vi "PathPlanner_Waypoint_AutoCtrlPoints.vi"(4 "NextExists":bool, 6 "PrevExists":bool, 8 "NextAnchor":T2 {"Y" format="%14.3f"; "X" format="%14.3f"}, 9 "PrevAnchor":T2 {"Y" format="%14.3f"; "X" format="%14.3f"}, 10 "Heading":T1={"VALUE"=0.0, "COS"=1.0, "SIN"=0.0} {"SIN" format="%13.4f"; "COS" format="%13.4f"; "VALUE" format="%13.4f"}, 11 "Anchor":T2 {"Y" format="%14.3f"; "X" format="%14.3f"}) -> (3 "Waypoint":T3 {"nextControl"."Y" format="%14.3f"; "nextControl"."X" format="%14.3f"; "anchor"."Y" format="%14.3f"; "anchor"."X" format="%14.3f"; "prevControl"."Y" format="%14.3f"; "prevControl"."X" format="%14.3f"})   [LabVIEW 2019, in "PathPlanner24.lvlib"]
doc: "Convert bezier points to waypoints allowing them to be written to a JSON string.\n\nInputs: \n - Bezier - array of translation2s - List of bezier points\n\nOutputs:\n - waypoints - array of cluster - waypoints compatible with pathplanner path JSON strings."
uses:
  PathPlanner24.lvlib
  TypeDef/PathPlannerWaypoint.ctl
  <vilib>/Rock Robotics/WPI/ThirdParty/JAS_Junk/TrajLib/TypeDef/TRANSLATION2D.ctl
  <vilib>/Rock Robotics/WPI/ThirdParty/JAS_Junk/TrajLib/Trajectory_Library.lvlib
  <vilib>/Rock Robotics/WPI/ThirdParty/JAS_Junk/TrajLib/TypeDef/ROTATION2D.ctl
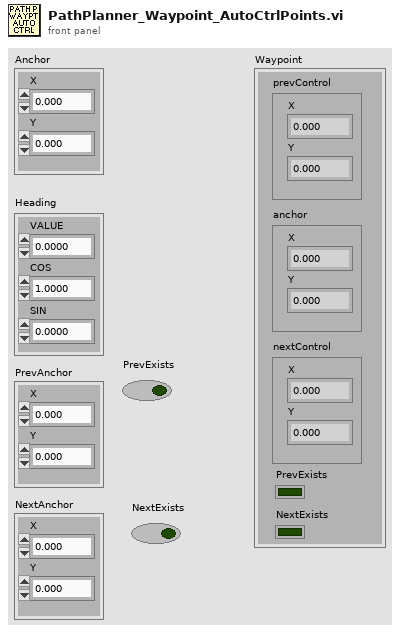
[diagram p1: front panel]
types:
  T1 = typedef "Trajectory_Library.lvlib/ROTATION2D.ctl" = cluster{"VALUE":dbl, "COS":dbl, "SIN":dbl}
  T2 = typedef "Trajectory_Library.lvlib/TRANSLATION2D.ctl" = cluster{"X":dbl, "Y":dbl}
  T3 = typedef "PathPlanner24.lvlib/PathPlannerWaypoint.ctl" = cluster{"prevControl":T2, "anchor":T2, "nextControl":T2, "PrevExists":bool, "NextExists":bool}
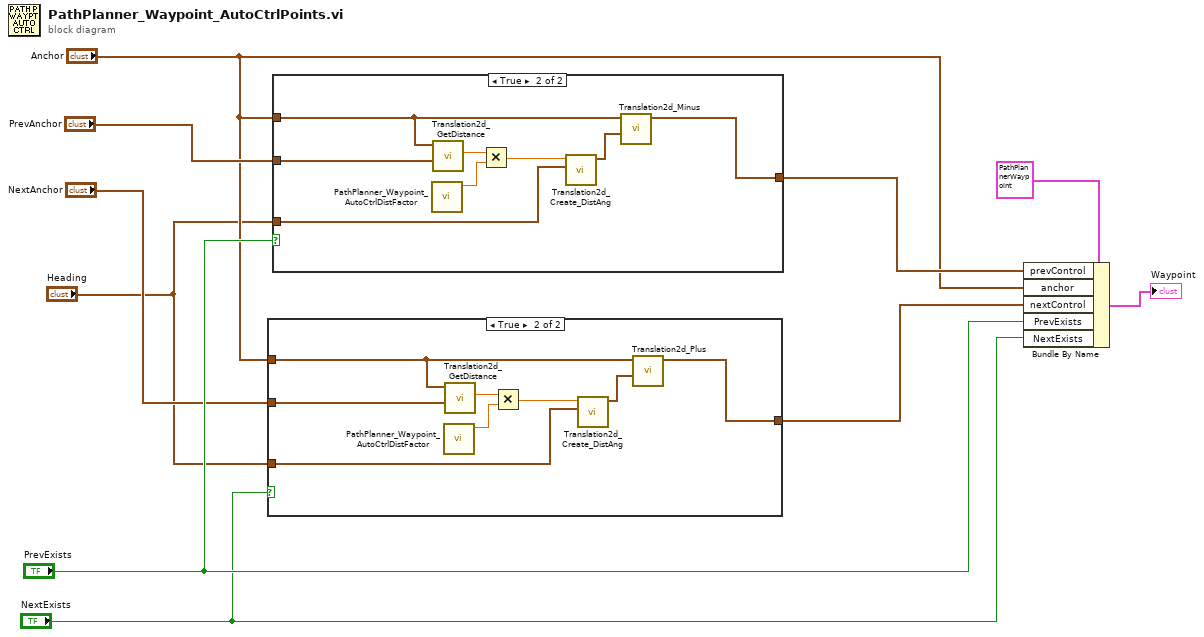
[diagram p0: block diagram]
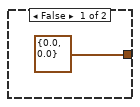
[diagram p2: hidden frame]
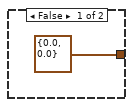
[diagram p3: hidden frame]
diagram:
  n1 = case shown="True" "NextExists" {
    tunnel: [T2 {"X"=0.0, "Y"=0.0} ("prevControl") w12] -> w5
    tunnel: "Anchor" -> [_ w15]
    tunnel: "NextAnchor" -> [_ w14]
    tunnel: "Heading" -> [_ w13]
    frame False {
    }
    frame True {
      n2 = call "PathPlanner_Waypoint_AutoCtrlDistFactor.vi"() -> ("AUTO_CONTROL_DISTANCE_FACTOR"=w17:dbl)  [unwired: 11 in]
      n3 = call <vilib>:"Translation2d_GetDistance.vi"("other Translation"=w14, "In Translation"=w15) -> ("Distance"=w18:dbl)  [unwired: 9 in]
      n4 = Multiply(x=w18, y=w17) -> (x*y=w16:dbl)
      n5 = call <vilib>:"Translation2d_Create_DistAng.vi"("Angle"=w13, "Dist"=w16) -> ("TRANSLATION"=w19:T2)  [unwired: 9 in]
      n6 = call <vilib>:"Translation2d_Plus.vi"("other Translation"=w19, "In Translation"=w15) -> ("Out Translation"=w12:T2)  [unwired: 9 in]
    }
  }
  n7 = case shown="True" "PrevExists" {
    tunnel: [T2 {"X"=0.0, "Y"=0.0} ("prevControl") w21] -> w6
    tunnel: "Anchor" -> [_ w26]
    tunnel: "Heading" -> [_ w27]
    tunnel: "PrevAnchor" -> [_ w25]
    frame False {
    }
    frame True {
      n8 = call "PathPlanner_Waypoint_AutoCtrlDistFactor.vi"() -> ("AUTO_CONTROL_DISTANCE_FACTOR"=w23:dbl)  [unwired: 11 in]
      n9 = call <vilib>:"Translation2d_GetDistance.vi"("other Translation"=w25, "In Translation"=w26) -> ("Distance"=w24:dbl)  [unwired: 9 in]
      n10 = Multiply(x=w24, y=w23) -> (x*y=w22:dbl)
      n11 = call <vilib>:"Translation2d_Create_DistAng.vi"("Angle"=w27, "Dist"=w22) -> ("TRANSLATION"=w28:T2)  [unwired: 9 in]
      n12 = call <vilib>:"Translation2d_Minus.vi"("other Translation"=w28, "In Translation"=w26) -> ("Out Translation"=w21:T2)  [unwired: 9 in]
    }
  }
  n13 = Bundle By Name(cluster=T3 {"prevControl"={"X"=0.0, "Y"=0.0}, "anchor"={"X"=0.0, "Y"=0.0}, "nextControl"={"X"=0.0, "Y"=0.0}, "PrevExists"=FALSE, "NextExists"=FALSE} ("Waypoint"), "prevControl"=w6, "anchor"="Anchor", "nextControl"=w5, "PrevExists"="PrevExists", "NextExists"="NextExists") -> (→"Waypoint":T3)
